vi "PlotData.vi"() -> ()   [LabVIEW 2013]
uses:
  <vilib>/Utility/file.llb/Read From Spreadsheet File (DBL).vi
panel:
  out "YArray 2":dbl[](array[numeric])
  out "XArray":dbl[](array[numeric])
  in  "# of sweeps":i32=1000
  out "Spectrum #":i32=999
  out "Chars":i32=1282716
  out "Fcen":dbl=213.0 format="%#_13g"
  out "# Data points":i32=81
  out "NMR Graph + Fit":cluster{dbl, dbl}[](graph)=[{212.8, -0.46521245828698476}, {212.805, -0.451738042269188}, {212.81, -0.4361992213570638}, {212.815, -0.423063070077864}, {212.82000000000002, -0.4129858731924357}, {212.82500000000002, -0.39950200222469395}, {212.83, -0.3896972191323693}, {212.835, -0.37960778642936577}, {212.84, -0.3704715239154619}, {212.845, -0.3613756395995548}, {212.85000000000002, -0.3542806451612908}, {212.85500000000002, -0.34573826473859853}, {212.86, -0.3389151279199112}, {212.865, -0.3356645161290327}, {212.87, -0.32928698553948893}, {212.875, -0.3245533926585096}, {212.88, -0.3195674082313677}, {212.88500000000002, -0.31636484983314794}, {212.89000000000001, -0.31329766407119025}, {212.895, -0.30928097886540584}, {212.9, -0.3076335928809786}, {212.905, -0.3051696329254729}, {212.91, -0.3036011123470524}, {212.915, -0.3027078976640709}, {212.92000000000002, -0.3008886540600665}, {212.925, -0.30022525027808694}, {212.93, -0.30038031145717464}, {212.935, -0.29949098998887647}, {212.94, -0.2997696329254728}, {212.945, -0.2997037819799777}, {212.95, -0.3008530589543934}, {212.955, -0.30116340378198003}, {212.96, -0.3008441601779759}, {212.965, -0.30301490545050047}, {212.97, -0.30069076751946616}, {212.975, -0.3028248053392658}, {212.98, -0.303430144605117}, {212.985, -0.30305194660734136}, {212.99, -0.30589265850945535}, {212.995, -0.30519688542825396}, {213.0, -0.30662758620689673}, {213.005, -0.30504037819799745}, {213.01, -0.3073824249165735}, {213.015, -0.30678731924360375}, {213.02, -0.3061101223581758}, {213.025, -0.30651223581757503}, {213.03, -0.3057032258064513}, {213.035, -0.3055011123470525}, {213.04, -0.3034794215795326}, {213.045, -0.3025264738598445}, {213.05, -0.29928598442714127}, {213.055, -0.2987539488320353}, {213.06, -0.2956502780867632}, {213.065, -0.2924911012235821}, {213.07, -0.28922858731924417}, {213.075, -0.2846795328142374}, {213.07999999999998, -0.2807577308120136}, {213.085, -0.2763669632925469}, {213.09, -0.2720147942157951}, {213.095, -0.26477352614015554}, {213.1, -0.2591063403781981}, {213.105, -0.250758954393771}, {213.10999999999999, -0.24276573971078985}, {213.11499999999998, -0.23413014460511672}, {213.12, -0.2249777530589542}, {213.125, -0.21574538375973307}, {213.13, -0.20545450500556167}, {213.135, -0.19439221357063405}, {213.14, -0.18102413793103433}, {213.14499999999998, -0.16831835372636259}, {213.14999999999998, -0.15441256952169063}, {213.155, -0.14002936596218032}, {213.16, -0.12397185761957694}, {213.165, -0.10871190211345938}, {213.17, -0.09141713014460523}, {213.17499999999998, -0.07229299221357056}, {213.17999999999998, -0.05475406006674076}, {213.185, -0.033457730812013316}, {213.19, -0.01384126807563961}, {213.195, 0.007918464961067835}, {213.2, 0.030717018909899838}]
  out "File size (bytes)":i32=1284000
  out "File name":string="C:\\Documents and Settings\\Patrick McGaughey\\Desktop\\rssmt\\NMR3489070215.xls"
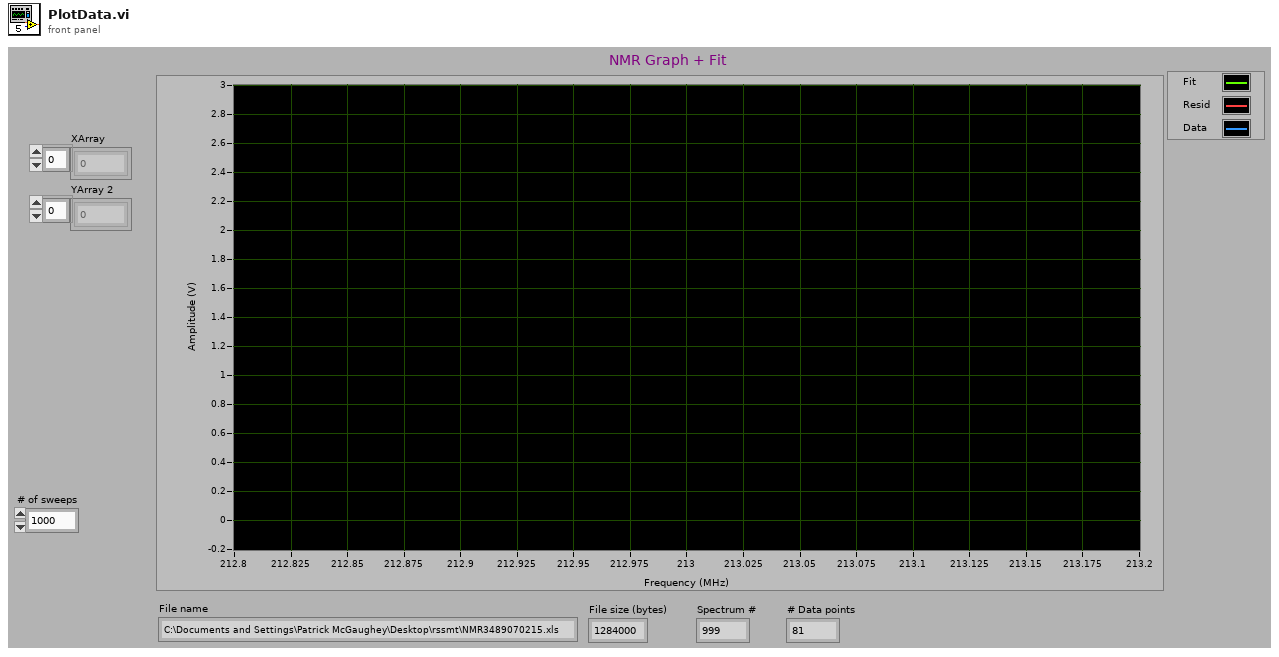
[diagram p1: front panel]
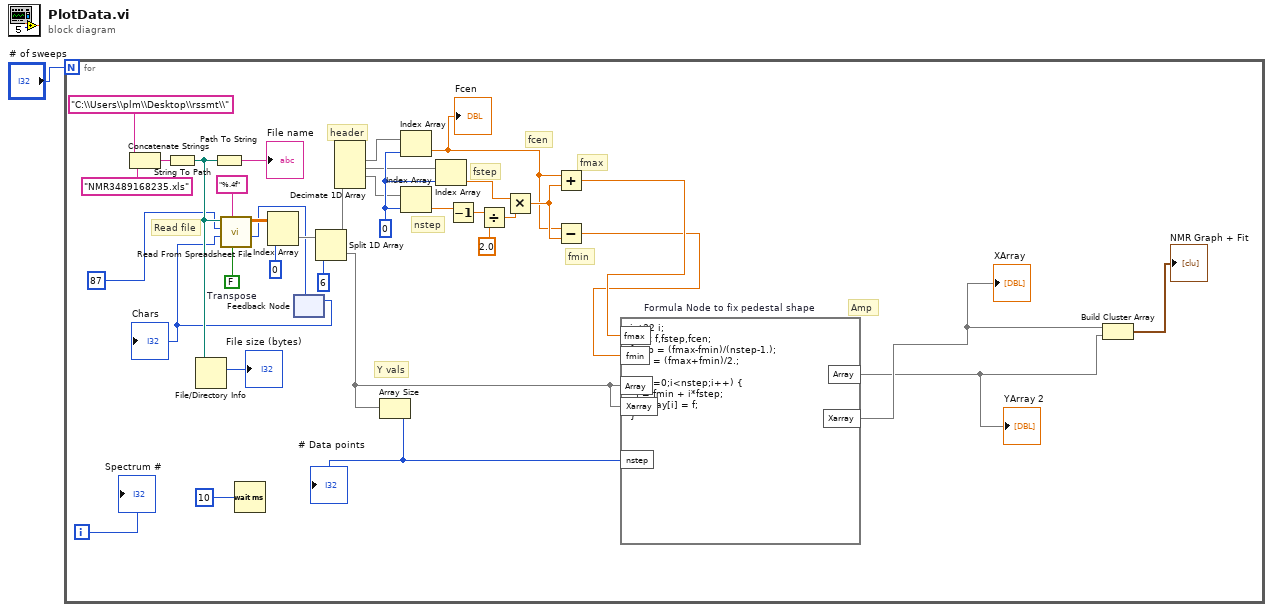
[diagram p0: block diagram]
diagram:
  n1 = for {
    N: "# of sweeps" -> [_]
    i -> [w8]
    w19 = 0
    w33 = FALSE  # Transpose
    # "Read file"
    # "header"
    # "nstep"
    # "fstep"
    # "fcen"
    # "fmin"
    # "fmax"
    # "Amp"
    # "Y vals"
    n2 = Concatenate Strings "Concatenate Strings"("C:\\Users\\plm\\Desktop\\rssmt\\", "NMR3489168235.xls") -> (w36:string)
    n3 = String To Path(string=w36) -> (path=w32:path)
    n4 = File/Directory Info(path=w32) -> (size=→"File size (bytes)":i64)  [unwired: 1 in, 6 out]
    n5 = Path To String(path=w32) -> (string=→"File name":string)
    n6 = Wait (ms)(milliseconds to wait=10) -> ()  [unwired: 1 out]
    n7 = feedback #1() -> (w10:i32)  [unwired: 1 in]
    "Chars" <- w10
    n8 = call-poly <vilib>:"Read From Spreadsheet File.vi"("transpose (no:F)"=w33, "format (%.3f)"="%.4f", "start of read offset (chars.:0)"=w10, "number of rows (all:-1)"=87, "file path (dialog if empty)"=w32) -> ("mark after read (chars.)"=w11:i32, "all rows"=w27:dbl[][])  [unwired: 2 in, 3 out]
    n9 = Index Array "Index Array"(array=w27, index (col)=0) -> (element=w25:dbl[])  [unwired: 1 in]
    n10 = feedback-in #1(w11) -> ()
    n11 = Split 1D Array(array=w25, index=6) -> (first subarray=w28:dbl[], second subarray=w4:dbl[])
    n12 = Decimate 1D Array(w28) -> (w20:dbl[], w18:dbl[], w17:dbl[])  [unwired: 3 out]
    n13 = Array Size(array=w4) -> (size(s)=w9:i32)
    "# Data points" <- w9
    n14 = Index Array "Index Array"(array=w20, index=w19) -> (element=w12:dbl)
    "Fcen" <- w12
    n15 = Index Array(array=w17, index=w19) -> (element=w15:dbl)
    n16 = Index Array(array=w18, index=w19) -> (element=w16:dbl)
    n17 = Decrement(x=w15) -> (x-1=w24:dbl)
    n18 = Divide(x=w24, y=2.0) -> (x/y=w22:dbl)
    n19 = Multiply(x=w16, y=w22) -> (x*y=w21:dbl)
    n20 = Add(x=w12, y=w21) -> (x+y=w6:dbl)
    n21 = Subtract(x=w12, y=w21) -> (x-y=w5:dbl)
    n22 = formula code="int32 i;\nfloat f,fstep,fcen;\nfstep = (fmax-fmin)/(nstep-1.);\nfcen = (fmax+fmin)/2.;\n\nfor (i=0;i<nstep;i++) {\n  f = fmin + i*fstep;\n  Xarray[i] = f;\n}" "Formula Node to fix pedestal shape"("nstep"=w9, "fmin"=w5, "fmax"=w6, "Array"=w4, "Xarray"=w4) -> ("Array"=w2:dbl[], "Xarray"=w3:dbl[])
    "XArray" <- w3
    "YArray 2" <- w2
    n23 = Build Cluster Array ("Index & Bundle Cluster Array")(w3, w2) -> (→"NMR Graph + Fit":cluster{dbl, dbl}[])
    "Spectrum #" <- w8
  }
